vi "InitTableFromDevices.vi"(6 "Defer Updates? (T)":bool=TRUE, 7 "Layout Ref":refnum<vi>, 8 "error in (no error)":errorcluster, 10 "Table Ref in":refnum<vi>, 11 "Devices queue":refnum<queue>) -> (0 "error out":errorcluster, 1 "Col array":refnum<class "Column.lvclass">[](array[class]), 2 "DevNums":i32[](array[numeric]), 3 "Devices queue out":refnum<queue>)   [LabVIEW 2013]
doc: "Initialize SetList Table from Device array. \"DevNums\" and \"Col array\" are output and must be set. Devices out only needs to be set if \"Devices in\" is empty.\n\nIf \"Devices in\" is empty, a master object (PulseBlaster) is initialized with a single row of default data and the \"default layout\" is added to the Layout ring. If \"Devices in\" is not empty, it is up to the programmer to make sure Layouts match the devices.\n\nEvidently, this VI needs write access to the Column array."
uses:
  ColumnVIs/Column/Column.lvclass
  Device/Device.lvclass
  Pulseblaster/Pulseblaster.lvclass
  Master Device/Master Device.lvclass
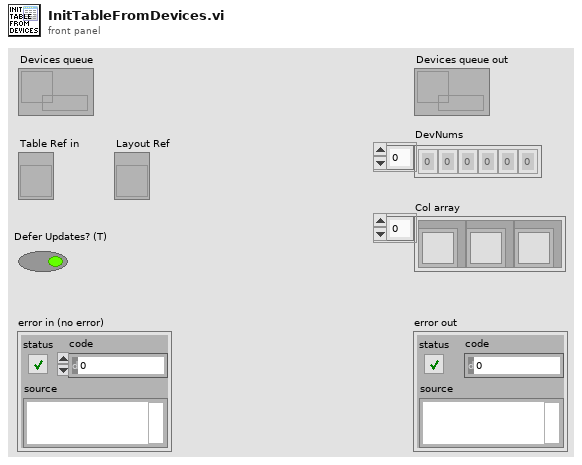
[diagram p1: front panel]
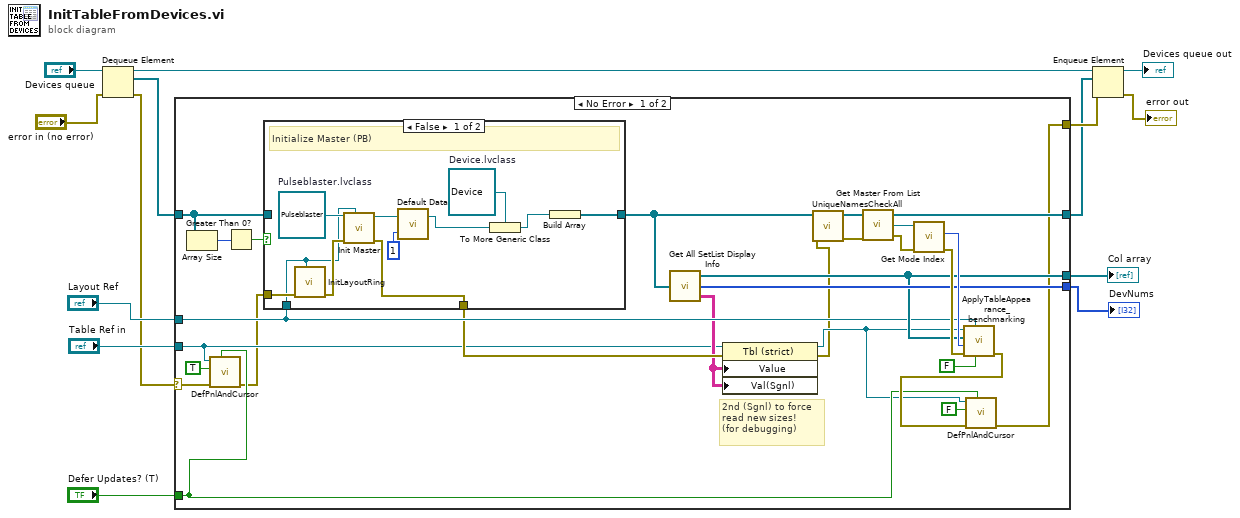
[diagram p0: block diagram]
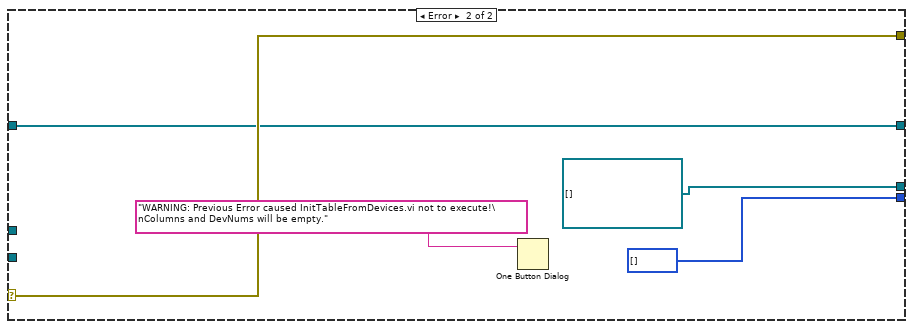
[diagram p3: hidden frame]
diagram:
  n1 = Dequeue Element(queue="Devices queue", error in (no error)="error in (no error)") -> (queue out=w8:refnum<queue>, element=w1:refnum<class "Device.lvclass">[], error out=w5:errorcluster)  [unwired: 1 in, 1 out]
  n2 = case shown="No Error" w5 {
    selector: w5 -> [w24 w59]
    tunnel: [w26 w59] -> w4
    tunnel: "Table Ref in" -> [w23 _]
    tunnel: "Defer Updates? (T)" -> [w21 _]
    tunnel: w1 -> [w41 w55]
    tunnel: [w40 w55] -> w2
    tunnel: [w35 i32[] [] ("DevNums")] -> w12
    tunnel: [w34 refnum<class "Column.lvclass">[] [] ("Columns")] -> w11
    tunnel: "Layout Ref" -> [w31 _]
    frame No Error {
      # "2nd (Sgnl) to force\nread new sizes!\n(for debugging)"
      n3 = Array Size(array=w41) -> (size(s)=w33:i32)
      n4 = call "DefPnlAndCursor.vi"("AllowDefPan? (T)"=w21, "error in (no error)"=w24, "DeferPanUpdts?"=TRUE, "Tbl Ctrl Refnum"=w23) -> ("error out"=w20:errorcluster)  [unwired: 7 in]
      n5 = Greater Than 0?(x=w33) -> (x > 0?=w32:bool)
      n6 = case shown="False" w32 {
        tunnel: w41 -> [_ w54]
        tunnel: [w47 w54] -> w18
        tunnel: w20 -> [w52 w53]
        tunnel: w31 -> [w42 _]
        tunnel: [w46 w53] -> w30
        frame False {
          w43 = refnum<class "Device.lvclass"> refnum  # Device.lvclass
          w51 = refnum<class "Pulseblaster.lvclass"> refnum  # Pulseblaster.lvclass
          # "Initialize Master (PB)"
          n7 = call "InitLayoutRing.vi"("Layouts Ring Refnum"=w42, "error in (no error)"=w52) -> ("error out"=w50:errorcluster)  [unwired: 9 in]
          n8 = call-dynamic "Init Master.vi"("Select Layout"=w42, "error in (no error)"=w50, "Pulseblaster in"=w51) -> ("error out"=w46:errorcluster, "Pulseblaster out"=w49:refnum<class "Pulseblaster.lvclass">)  [unwired: 7 in]
          n9 = call-dynamic "Default Data.vi"("Num Rows"=1, "Pulseblaster in"=w49) -> ("Pulseblaster out"=w45:refnum<class "Pulseblaster.lvclass">)  [unwired: 1 out]
          n10 = To More Generic Class(target class=w43, reference=w45) -> (generic class reference=w44:refnum<class "Device.lvclass">)
          n11 = Build Array(w44) -> (w47:refnum<class "Device.lvclass">[])
        }
        frame True {
          # "Device array has elements"
        }
      }
      n12 = call "Get All SetList Display Info.vi"("Devices"=w18) -> ("Columns"=w34:refnum<class "Column.lvclass">[], "DevNums"=w35:i32[], "Table Data"=w29:string[][])
      n13 = property on="Property Node" class="Tbl (strict)"(reference=w23, error in=w30, "Value"=w29, "Val(Sgnl)"=w29) -> (reference out=w19:refnum<vi>, error out=w16:errorcluster)
      n14 = call "UniqueNamesCheckAll.vi"("error in (no error)"=w16, "Devices"=w18) -> ("error out"=w15:errorcluster, "Devices out"=w17:refnum<class "Device.lvclass">[])  [unwired: 8 in]
      n15 = call "Get Master From List.vi"("error in"=w15, "Device List in"=w17) -> ("error out"=w38:errorcluster, "Master Device"=w39:refnum<class "Master Device.lvclass">, "Device List out"=w40:refnum<class "Device.lvclass">[])  [unwired: 1 in]
      n16 = call-dynamic "Get Mode Index.vi"("error in (no error)"=w38, "Master Device in"=w39) -> ("error out"=w37:errorcluster, "Mode Col"=w36:i32)  [unwired: 7 in, 1 out]
      n17 = call "ApplyTableAppearance_benchmarking.vi"("Defer Updates? (T)"=FALSE, "Layout Ring Ref"=w31, "error in (no error)"=w37, "Mode Index"=w36, "Col Array in"=w34, "Table Ref in"=w19) -> ("error out"=w27:errorcluster)  [unwired: 4 in, 1 out]
      n18 = call "DefPnlAndCursor.vi"("AllowDefPan? (T)"=w21, "error in (no error)"=w27, "DeferPanUpdts?"=FALSE, "Tbl Ctrl Refnum"=w19) -> ("error out"=w26:errorcluster)  [unwired: 7 in]
    }
    frame Error {
      n19 = One Button Dialog(message="WARNING: Previous Error caused InitTableFromDevices.vi not to execute!\nColumns and DevNums will be empty.") -> ()  [unwired: 1 in, 1 out]
    }
  }
  "DevNums" <- w12
  "Col array" <- w11
  n20 = Enqueue Element(queue=w8, element=w2, error in (no error)=w4) -> (queue out=→"Devices queue out":refnum<queue>, error out=→"error out":errorcluster)  [unwired: 1 in, 1 out]
